vi "Add Endpoint.vi"(5 "Template (\"\"=Static File)":string, 6 "Replace if exists? (T)":bool=TRUE, 7 "VI Refnum in":refnum<vi>, 8 "error in (no error)":errorcluster, 9 "Content-Type":string, 10 "Content":string, 11 "Endpoint":string) -> (0 "error out":errorcluster, 1 "Created?":bool)   [LabVIEW 2021, in "HttpServer.lvlib"]
uses:
  HttpServer.lvlib
  TypeDefs/Action.ctl
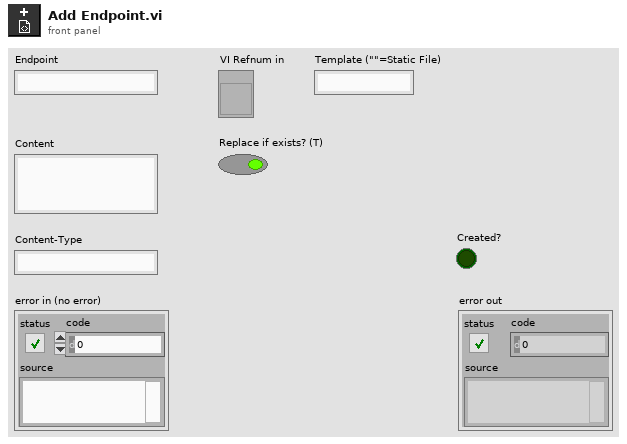
[diagram p1: front panel]
types:
  T1 = typedef "HttpServer.lvlib/Action.ctl" = enum8{"noop", "add", "get", "set", "remove"}
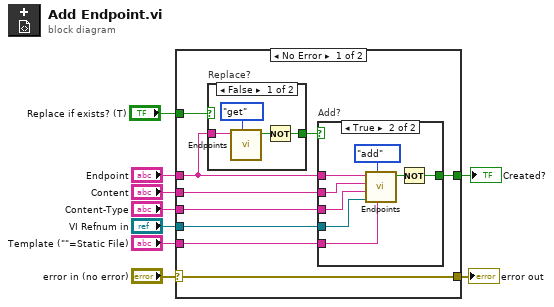
[diagram p0: block diagram]
diagram:
  n1 = case shown="No Error" "error in (no error)" {
    selector: "error in (no error)" -> [w15 w32]
    tunnel: "Endpoint" -> [w14 _]
    tunnel: "Content" -> [w18 _]
    tunnel: "Content-Type" -> [w17 _]
    tunnel: "VI Refnum in" -> [w16 _]
    tunnel: [w15 w32] -> w5
    tunnel: "Replace if exists? (T)" -> [w13 _]
    tunnel: [w11 _] -> w2
    tunnel: "Template (\"\"=Static File)" -> [w10 _]
    frame No Error {
      n2 = case "Replace?" shown="False" w13 {
        selector: w13 -> [_ w23]
        tunnel: w14 -> [w21 _]
        tunnel: [w19 w23] -> w12
        frame False {
          n3 = call "Endpoints.vi"("Action"=Action."get", "Endpoint"=w21) -> ("Found?"=w20:bool)  [unwired: 4 in, 5 out]
          n4 = Not(x=w20) -> (.not. x?=w19:bool)
        }
        frame True {
        }
      }
      n5 = case "Add?" shown="True" w12 {
        tunnel: w18 -> [_ w30]
        tunnel: w17 -> [_ w29]
        tunnel: w16 -> [_ w28]
        tunnel: w14 -> [_ w27]
        tunnel: [_ w25] -> w11
        tunnel: w10 -> [_ w24]
        frame False {
        }
        frame True {
          n6 = call "Endpoints.vi"("Template in"=w24, "Action"=Action."add", "VI Refnum in"=w28, "Content-Type in"=w29, "Content in"=w30, "Endpoint"=w27) -> ("Found?"=w26:bool)  [unwired: 5 out]
          n7 = Not(x=w26) -> (.not. x?=w25:bool)
        }
      }
    }
    frame Error {
    }
  }
  "error out" <- w5
  "Created?" <- w2
